vi "BPSK_Filtering.vi"(5 "UpSampleRate":dbl, 8 "error in (no error)":errorcluster caption="错误输入（无错误）", 10 "input_data":dbl[](array[numeric]) format="%#_13g", 11 "PathIn":path) -> (0 "error out":errorcluster caption="错误输出", 2 "out_data":dbl[](array[numeric]), 3 "PathOut":path)   [LabVIEW 2015]
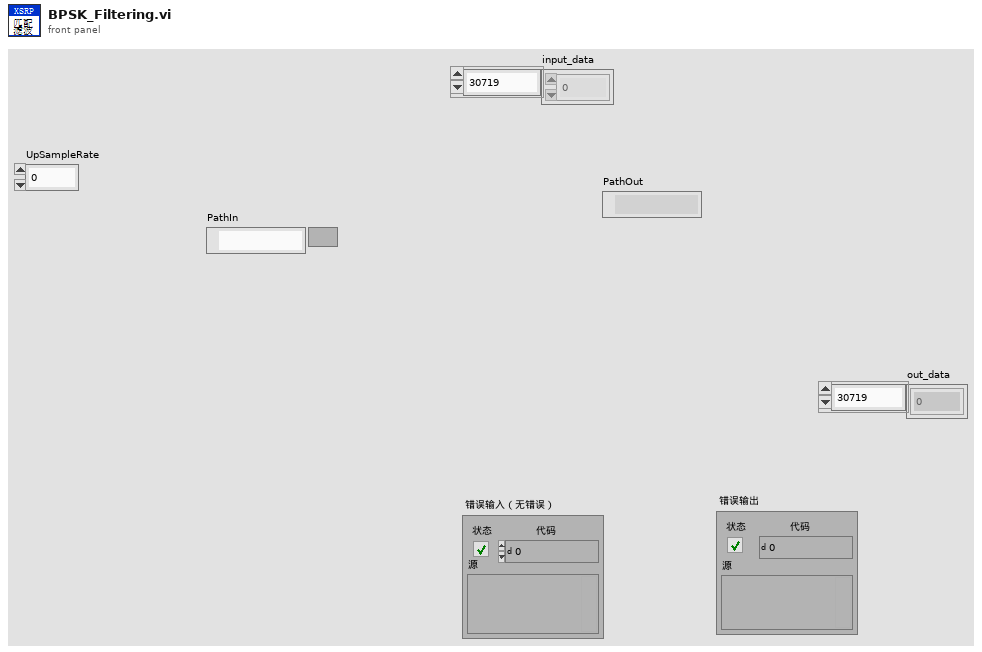
[diagram p1: front panel]
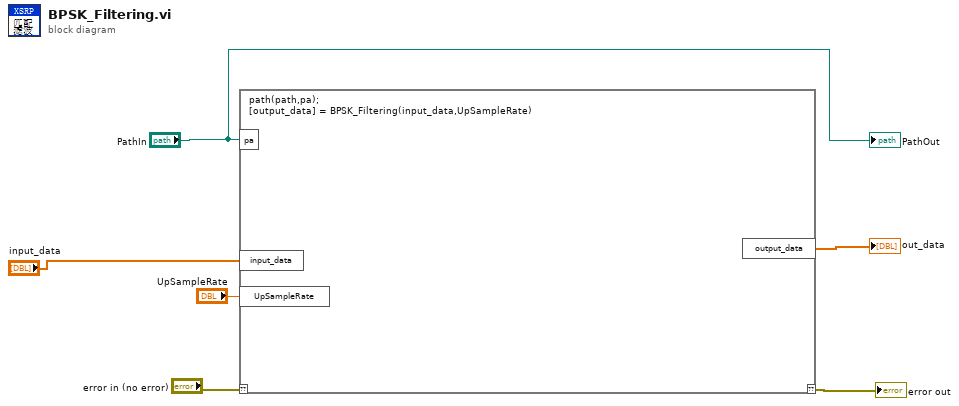
[diagram p0: block diagram]
diagram:
  n1 = script code="path(path,pa);\n[output_data] = BPSK_Filtering(input_data,UpSampleRate)"("??"="error in (no error)", "pa"="PathIn", "input_data"="input_data", "UpSampleRate"="UpSampleRate") -> ("??"=→"error out":errorcluster, "output_data"=→"out_data":dbl[])
  "PathOut" <- "PathIn"
